vi "Module_Initialize_SMU's.vi"(8 "Error In":errorcluster, 11 "Instrument_Visas":T1) -> (0 "Error Out":errorcluster)   [LabVIEW 2013]
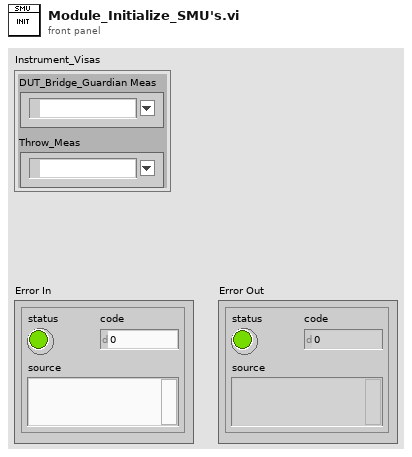
[diagram p1: front panel]
types:
  T1 = cluster{"DUT_Bridge_Guardian Meas":refnum<k15>, "Throw_Meas":refnum<k15>}
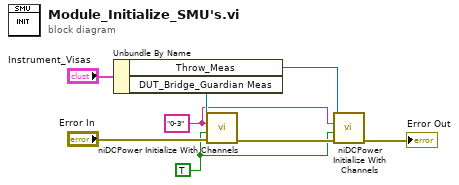
[diagram p0: block diagram]
diagram:
  w1 = TRUE ("reset (false)")
  w3 = "0-3" ("channels")
  n1 = Unbundle By Name("Instrument_Visas") -> ("Throw_Meas"=w2:refnum<k15>, "DUT_Bridge_Guardian Meas"=w7:refnum<k15>)
  n2 = call <instrlib>:"niDCPower Initialize With Channels.vi"("error in (no error)"="Error In", "reset (false)"=w1, "channels"=w3, "resource name"=w7) -> ("error out"=w5:errorcluster)  [unwired: 6 in, 1 out]
  n3 = call <instrlib>:"niDCPower Initialize With Channels.vi"("error in (no error)"=w5, "reset (false)"=w1, "channels"=w3, "resource name"=w2) -> ("error out"=→"Error Out":errorcluster)  [unwired: 6 in, 1 out]
